vi "Stop Core.vi"(10 "final error code":i32, 11 "Measure Object in":refnum<class "TCP Communications.lvclass">) -> (3 "Measure Object out":refnum<class "TCP Communications.lvclass">)   [LabVIEW 2016, in "TCP Communications.lvclass"]
doc: "(<B>Filename</B>: Actor Framework.lvlib:Actor.lvclass:Stop Core.vi)\n\nDefines what the actor does before it stops. Use the <B>final error code</B> input to determine whether the actor shut down in response to an error.\n\nBy default, this method does nothing. A descendant class may override it to define behavior, such as shutting down any processes the actor initiated in its override of the Actor Core method."
uses:
  TCP Communications.lvclass
  TCP Communications.lvclass/TCP Communications.ctl
  Communications/Communications.lvclass
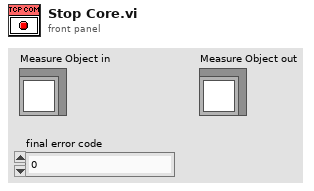
[diagram p1: front panel]
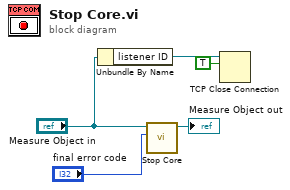
[diagram p0: block diagram]
diagram:
  n1 = Unbundle By Name("Measure Object in") -> ("listener ID"=w2:refnum<k5>)
  n2 = call-parent "Stop Core.vi"("final error code"="final error code", "Measure Object in"="Measure Object in") -> ("Measure Object out"=→"Measure Object out":refnum<class "TCP Communications.lvclass">)  [unwired: 9 in]
  n3 = TCP Close Connection(connection ID=w2, abort (F)=TRUE) -> ()  [unwired: 1 in, 2 out]
